vi "Draw Caster Wheel.vi"(6 "wheel state":T1, 7 "picture info":T3={"picture size"={"Width"=500, "Height"=500}, "pixels per unit"=10.0}, 8 "error in (no error)":errorcluster, 9 "draw wheel options":T2={"global wheel position"={"x"=0.0, "y"=0.0}, "wheel frame angle (rad)"=0.0, "color (black)"=0, "draw wheel state"=FALSE, "draw forward velocity"=FALSE, "velocity scale"=16711680.0, "velocity color (red)"=16711680}, 10 "picture in":picture, 11 "wheel in":refnum<class "NI_Robotics_Wheel.lvclass">) -> (0 "error out":errorcluster, 2 "picture out":picture, 3 "wheel out":refnum<class "NI_Robotics_Wheel.lvclass">)   [LabVIEW 2017, in "NI_Robotics_Steering Picture.lvlib"]
uses:
  <vilib>/robotics/Utilities/Visualization/Steering Visualization/Steering Picture/NI_Robotics_Steering Picture.lvlib
  <vilib>/robotics/Steering/Wheel/NI_Robotics_Wheel.lvclass
  <vilib>/robotics/Utilities/Visualization/Steering Visualization/Steering Picture/Picture Info.ctl
  <vilib>/Utility/miscctls.llb/LVBoundsTypeDef.ctl
  <vilib>/robotics/Utilities/Visualization/Steering Visualization/Steering Picture/Draw Wheel Options.ctl
  <vilib>/robotics/Steering/Wheel/Wheel State.ctl
  <vilib>/Analysis/coordinate.llb/2D Cartesian Coordinate Rotation (Scalar).vi
  <vilib>/Analysis/coordinate.llb/Angle Rotation (scalar).vi
  <vilib>/Analysis/coordinate.llb/2D Cartesian Coordinate Rotation (Array).vi
  <vilib>/Analysis/coordinate.llb/Wrap Angle (scalar).vi
  <vilib>/picture/picture.llb/Move Pen.vi
  <vilib>/robotics/Steering/Wheel/Get Caster Wheel Information.vi
  <vilib>/picture/picture.llb/Draw Multiple Lines.vi
  <vilib>/Analysis/NI_AALPro.lvlib
  <vilib>/Analysis/NI_AAL_Angle.lvlib
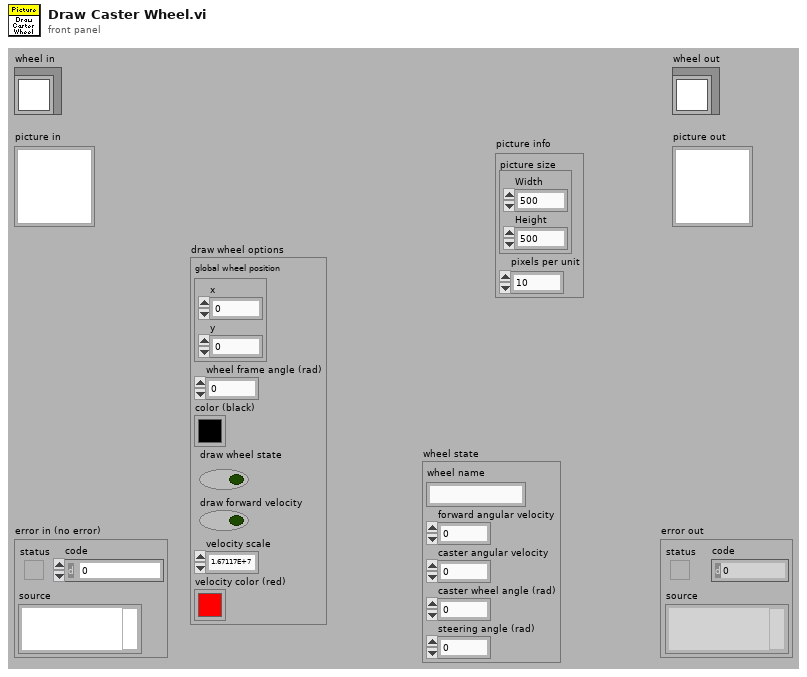
[diagram p1: front panel]
types:
  T1 = typedef "NI_Robotics_Wheel.lvclass/Wheel State.ctl" = cluster{"wheel name":string, "forward angular velocity":dbl, "caster angular velocity":dbl, "caster wheel angle (rad)":dbl, "steering angle (rad)":dbl}
  T2 = typedef "NI_Robotics_Steering Picture.lvlib/Draw Wheel Options.ctl" = cluster{"global wheel position":cluster{"x":dbl, "y":dbl}, "wheel frame angle (rad)":dbl, "color (black)":u32, "draw wheel state":bool, "draw forward velocity":bool, "velocity scale":dbl, "velocity color (red)":u32}
  T3 = typedef "NI_Robotics_Steering Picture.lvlib/Picture Info.ctl" = cluster{"picture size":T4, "pixels per unit":dbl}
  T4 = typedef "LVBoundsTypeDef.ctl" = cluster{"Width":u32, "Height":u32}
  T5 = cluster{"Width":u16, "Style":enum32{"Solid", "Dash", "Dot", "DashDot", "DashDotDot"}}
  T6 = typedef "NI_Robotics_Wheel.lvclass/Wheel Parameters.ctl" = cluster{"wheel radius":dbl, "gear ratio":dbl, "forward rotation direction":T7}
  T7 = typedef "NI_Robotics_Wheel.lvclass/Rotation Direction.ctl" = u16
  T8 = typedef "NI_Robotics_Caster Wheel.lvclass/Caster Wheel Parameters.ctl" = cluster{"forward offset":dbl, "caster gear ratio":dbl}
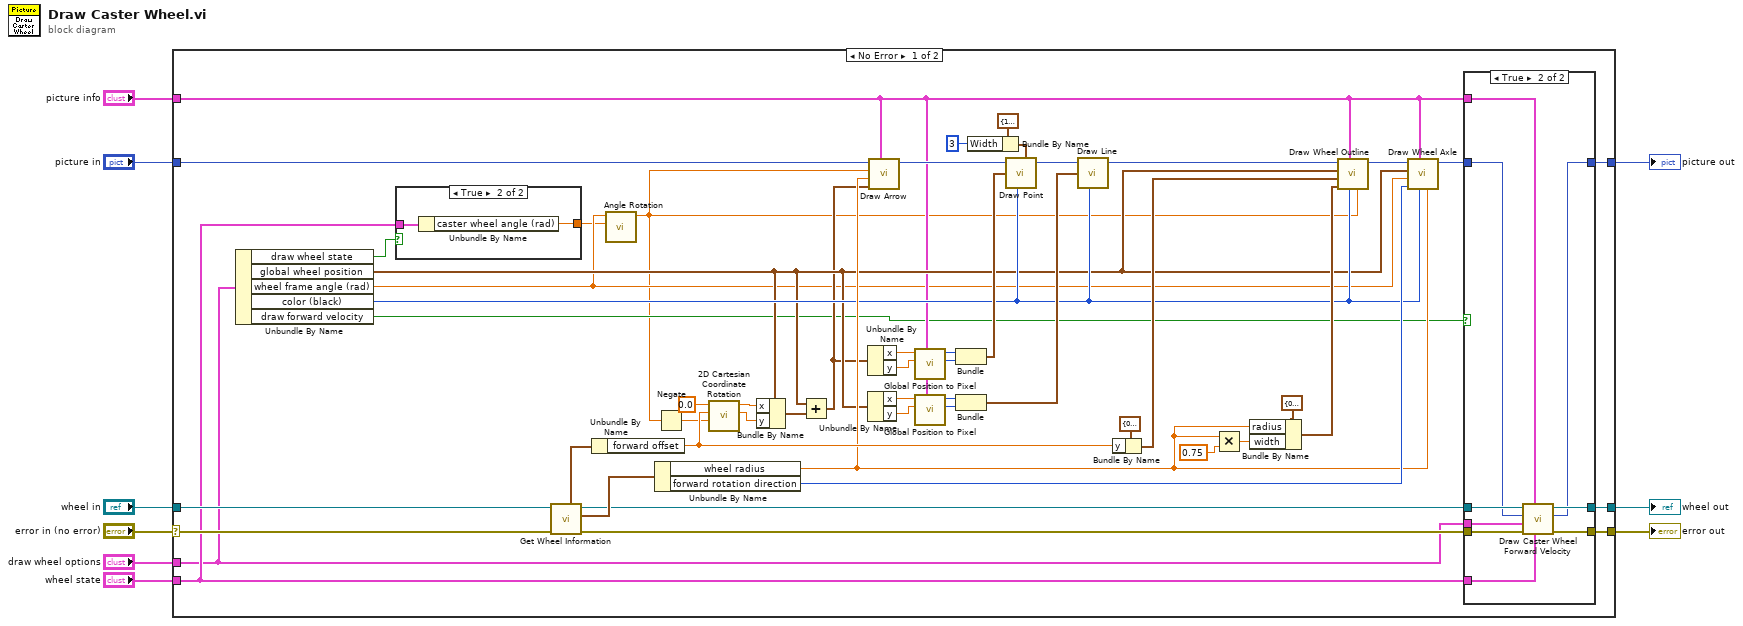
[diagram p0: block diagram]
diagram:
  n1 = case shown="No Error" "error in (no error)" {
    selector: "error in (no error)" -> [w61 w79]
    tunnel: [w20 w79] -> w8
    tunnel: "wheel in" -> [w62 w77]
    tunnel: "picture in" -> [w59 w78]
    tunnel: [w18 w78] -> w5
    tunnel: [w22 w77] -> w4
    tunnel: "picture info" -> [w17 _]
    tunnel: "draw wheel options" -> [w13 _]
    tunnel: "wheel state" -> [w14 _]
    frame No Error {
      n2 = Unbundle By Name(w13) -> ("draw wheel state"=w15:bool, "global wheel position"=w25:cluster{"x":dbl, "y":dbl}, "wheel frame angle (rad)"=w12:dbl, "color (black)"=w26:u32, "draw forward velocity"=w16:bool)
      n3 = case shown="True" w15 {
        tunnel: w14 -> [_ w64]
        tunnel: [_ w63] -> w10
        frame False {
        }
        frame True {
          n4 = Unbundle By Name(w64) -> ("caster wheel angle (rad)"=w63:dbl)
        }
      }
      n5 = call-poly <vilib>:"Get Wheel Information.vi"("error in (no error)"=w61, "wheel in"=w62) -> ("error out"=w21:errorcluster, "wheel parameters"=w58:T6, "wheel out"=w23:refnum<class "NI_Robotics_Wheel.lvclass">, "caster parameters"=w60:T8)  [unwired: 3 in, 3 out]
      n6 = Unbundle By Name(w60) -> ("forward offset"=w46:dbl)
      n7 = call-poly <vilib>:"Angle Rotation.vi"("counterclockwise rotation"=w10, "angle"=w12) -> ("rotated angle"=w11:dbl)  [unwired: 8 in, 1 out]
      n8 = Unbundle By Name(w58) -> ("wheel radius"=w27:dbl, "forward rotation direction"=w47:T7)
      n9 = Negate(x=w11) -> (-x=w44:dbl)
      n10 = call-poly <vilib>:"2D Cartesian Coordinate Rotation.vi"("theta"=w44, "y"=w46, "x"=0.0) -> ("y out"=w42:dbl, "x out"=w43:dbl)  [unwired: 6 in, 1 out]
      n11 = Bundle By Name(cluster=w25, "x"=w43, "y"=w42) -> (w41:cluster{"x":dbl, "y":dbl})
      n12 = Add(x=w25, y=w41) -> (x+y=w24:cluster{"x":dbl, "y":dbl})
      n13 = Unbundle By Name(w24) -> ("x"=w39:dbl, "y"=w38:dbl)
      n14 = Unbundle By Name(w25) -> ("x"=w30:dbl, "y"=w31:dbl)
      n15 = call <vilib>:"Draw Arrow.vi"("picture info"=w17, "global base position"=w24, "length"=w27, "wheel frame angle (rad)"=w11, "picture in"=w59) -> ("picture out"=w40:picture)  [unwired: 6 in]
      n16 = call <vilib>:"Global Position to Pixel.vi"("picture info"=w17, "global y"=w38, "global x"=w39) -> ("pixel y"=w36:i16, "pixel x"=w37:i16)  [unwired: 7 in]
      n17 = call <vilib>:"Global Position to Pixel.vi"("picture info"=w17, "global y"=w31, "global x"=w30) -> ("pixel y"=w33:i16, "pixel x"=w32:i16)  [unwired: 7 in]
      n18 = Bundle("pixel x"=w37, "pixel y"=w36) -> (w28:cluster{"pixel x":i16, "pixel y":i16})  [unwired: 1 in]
      n19 = Bundle("pixel x"=w32, "pixel y"=w33) -> (w29:cluster{"pixel x":i16, "pixel y":i16})  [unwired: 1 in]
      n20 = Bundle By Name(cluster=T5 {"Width"=1, "Style"=enum."Solid"} ("pen"), "Width"=u16 3) -> (w55:T5)
      n21 = call <vilib>:"Draw Point.vi"("picture"=w40, "point(x,y)"=w28, "color(black)"=w26, "pen"=w55) -> ("new picture"=w35:picture)  [unwired: 5 in]
      n22 = call <vilib>:"Draw Line.vi"("picture"=w35, "end point"=w29, "color(black)"=w26) -> ("new picture"=w34:picture)  [unwired: 6 in]
      n23 = Bundle By Name(cluster=cluster{"x":dbl, "y":dbl} {"x"=0.0, "y"=0.0} ("offset from center"), "y"=w46) -> (w53:cluster{"x":dbl, "y":dbl})
      n24 = Multiply(x=w27, y=0.75) -> (x*y=w49:dbl)
      n25 = Bundle By Name(cluster=cluster{"radius":dbl, "width":dbl} {"radius"=0.0, "width"=0.0} ("size"), "radius"=w27, "width"=w49) -> (w51:cluster{"radius":dbl, "width":dbl})
      n26 = call <vilib>:"Draw Wheel Outline.vi"("angle (rad)"=w11, "color (black)"=w26, "picture info"=w17, "size"=w51, "offset from center"=w53, "global wheel position"=w25, "picture in"=w34) -> ("picture out"=w48:picture)  [unwired: 4 in]
      n27 = call <vilib>:"Draw Wheel Axle.vi"("length"=w27, "color (black)"=w26, "picture info"=w17, "rotation direction"=w47, "wheel frame angle (rad)"=w12, "global wheel position"=w25, "picture in"=w48) -> ("picture out"=w19:picture)  [unwired: 4 in]
      n28 = case shown="True" w16 {
        tunnel: w23 -> [w66 w76]
        tunnel: [w66 w75] -> w22
        tunnel: w21 -> [w65 w74]
        tunnel: [w65 w73] -> w20
        tunnel: w19 -> [w67 w72]
        tunnel: [w67 w71] -> w18
        tunnel: w17 -> [_ w70]
        tunnel: w14 -> [_ w69]
        tunnel: w13 -> [_ w68]
        frame False {
        }
        frame True {
          n29 = call <vilib>:"Draw Caster Wheel Forward Velocity.vi"("wheel state"=w69, "picture info"=w70, "error in (no error)"=w74, "draw wheel options"=w68, "picture in"=w72, "wheel in"=w76) -> ("error out"=w73:errorcluster, "picture out"=w71:picture, "wheel out"=w75:refnum<class "NI_Robotics_Wheel.lvclass">)  [unwired: 3 in]
        }
      }
    }
    frame Error {
    }
  }
  "error out" <- w8
  "wheel out" <- w4
  "picture out" <- w5
